vi "Open Typedef.vi"(7 "App":refnum<vi>, 8 "error in (no error)":errorcluster, 11 "Typedef Path":path) -> (0 "error out":errorcluster, 2 "Control":refnum<vi>, 3 "VI":refnum<vi>)   [LabVIEW 2020, in "LV-Protoc.lvlib"]
uses:
  LV-Protoc.lvlib
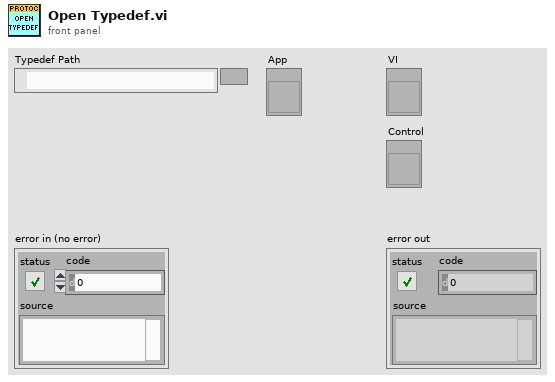
[diagram p1: front panel]
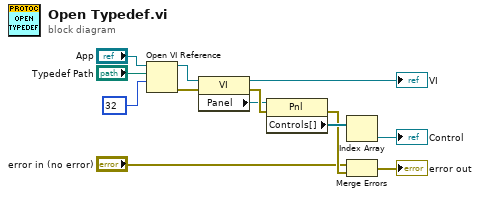
[diagram p0: block diagram]
diagram:
  n1 = Open VI Reference(application reference (local)="App", vi path="Typedef Path", options=32) -> (vi reference=w10:refnum<vi>, error out=w11:errorcluster)  [unwired: 3 in]
  n2 = property class="VI"(reference=w10, error in=w11) -> (reference out=→"VI":refnum<vi>, error out=w13:errorcluster, "Panel"=w9:refnum<vi>)
  n3 = property class="Pnl"(reference=w9, error in=w13) -> (error out=w4:errorcluster, "Controls[]"=w8:refnum<vi>[])  [unwired: 1 out]
  n4 = Index Array(array=w8) -> (element=→"Control":refnum<vi>)  [unwired: 1 in]
  n5 = Merge Errors("error in (no error)", w4) -> (→"error out":errorcluster)
